vi "Set_Parameters_Reference.vi"(8 "error in (no error)":errorcluster, 10 "Parameters_Reference":dbl[](array[numeric]), 11 "ExampleStateMachine runtime_in":refnum<class "ExampleStateMachine runtime.lvclass">) -> (0 "error out":errorcluster, 3 "ExampleStateMachine runtime_out":refnum<class "ExampleStateMachine runtime.lvclass">)   [LabVIEW 2017, in "ExampleStateMachine runtime.lvclass"]
uses:
  ExampleStateMachine runtime.lvclass
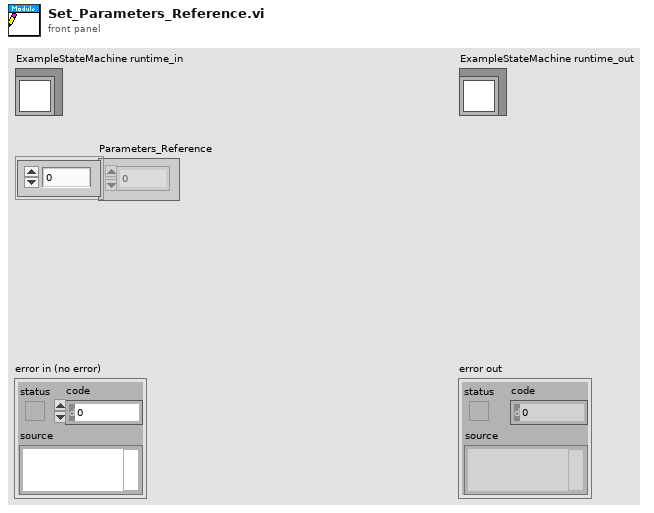
[diagram p1: front panel]
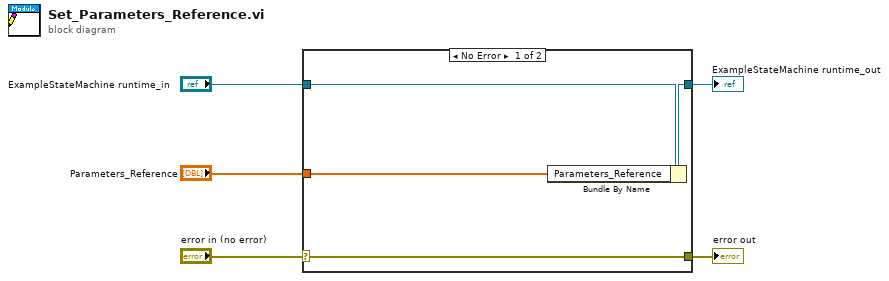
[diagram p0: block diagram]
diagram:
  n1 = case shown="No Error" "error in (no error)" {
    selector: "error in (no error)" -> [w9 w10]
    tunnel: [w9 w10] -> w4
    tunnel: [w7 w11] -> w2
    tunnel: "ExampleStateMachine runtime_in" -> [w8 w11]
    tunnel: "Parameters_Reference" -> [w6 _]
    frame No Error {
      n2 = Bundle By Name(cluster=w8, "Parameters_Reference"=w6) -> (w7:refnum<class "ExampleStateMachine runtime.lvclass">)
    }
    frame Error {
    }
  }
  "error out" <- w4
  "ExampleStateMachine runtime_out" <- w2
